vi "PH_PILS.set i Attr.vi"(2 "error in (no error)":errorcluster, 3 "DB Entry to read":string) -> (0 "error out":errorcluster, 1 "i Attr":T1={"Boolean"=[], "GUI Refs Exp. Shutters"={"1"=refnum, "2"=refnum, "3"=refnum, "4"=refnum}, "Tristate2Run GUI Refs"=[], "EO-Likes"=[], "Operation Mode"={"Operation Mode"=enum."unknown", "GUI"={"Ref State"=refnum, "Ref"=refnum}, "Servicemode"={"Tagname"="", "Status"=0}, "Labormode"={"Tagname"="", "Status"=0}, "Searchmode"={"Tagname"="", "Status"=0}, "Shotmode"={"Tagname"="", "Status"=0}}, "Submode"={"Submode"=enum."unknown", "GUI"={"Ref State"=refnum, "Ref"=refnum}, "Submode"={"Tagname"="", "Status"=0}}, "Experiment"={"Experiment"=enum."unknown", "GUI"={"Ref State"=refnum, "Ref"=refnum}, "intern"={"Tagname"="", "Status"=0}, "Exp 4"={"Tagname"="", "Status"=0}, "Exp 3"={"Tagname"="", "Status"=0}, "Exp 2"={"Tagname"="", "Status"=0}, "Exp 1"={"Tagname"="", "Status"=0}}, "TristateNormal"=[], "Door Tags"=[], "GUIlessTags"=[], "Beamline GUI Refs"=[], "Special Boolean"=[], "Laserpower"=[], "Shutter"=[], "Tristate EO Like"=[], "PP"=[], "Switch Knobs"=[], "Latch Knob GUI Refs"=[], "FailureCounter"=0, "Enabled Status"={"Laser"=0, "PreAmp"=0, "MainAmp"=0}, "Mercury"=refnum, "Instance Rods"="N/A", "Logfile"=path "", "Beckhoff-Instance Internal"="", "Beckhoff-Instance External"="", "Enabling Rights"=[]})   [LabVIEW 2014, in "PH_PILS.lvlib"]
doc: "This VI sets attributes."
uses:
  PH_PILS.lvlib
  PH_PILS.i attribute.ctl
  PH_PILS.Operation Mode.ctl
  PH_PILS.Submode.ctl
  PH_Common/PH_Common.lvlib
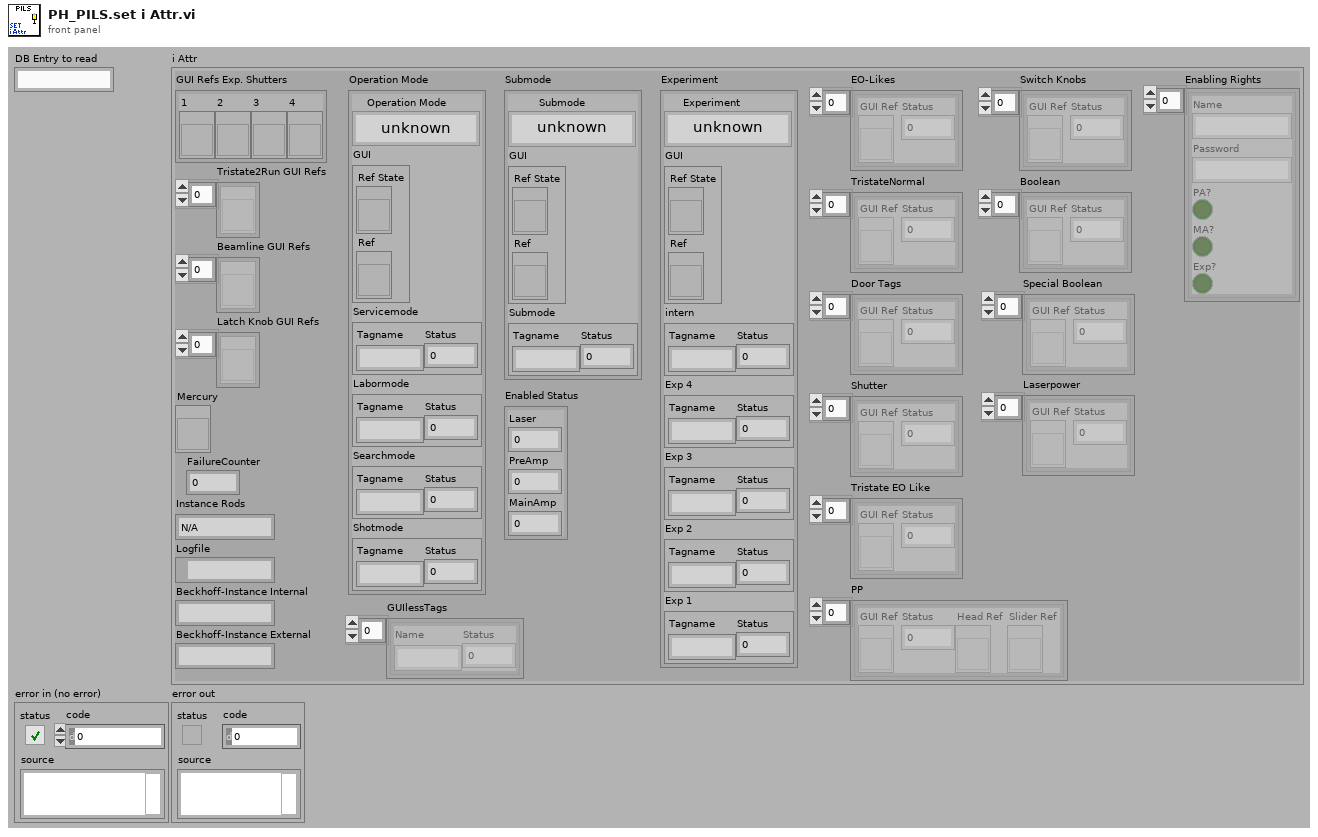
[diagram p1: front panel]
types:
  T1 = typedef "PH_PILS.lvlib/PH_PILS.i attribute.ctl" = cluster{"Boolean":cluster{"GUI Ref":refnum<vi>, "Status":i32}[], "GUI Refs Exp. Shutters":cluster{"1":refnum<vi>, "2":refnum<vi>, "3":refnum<vi>, "4":refnum<vi>}, "Tristate2Run GUI Refs":refnum<vi>[], "EO-Likes":cluster{"GUI Ref":refnum<vi>, "Status":i32}[], "Operation Mode":cluster{"Operation Mode":T2, "GUI":cluster{"Ref State":refnum<vi>, "Ref":refnum<vi>}, "Servicemode":cluster{"Tagname":string, "Status":i32}, "Labormode":cluster{"Tagname":string, "Status":i32}, "Searchmode":cluster{"Tagname":string, "Status":i32}, "Shotmode":cluster{"Tagname":string, "Status":i32}}, "Submode":cluster{"Submode":T3, "GUI":cluster{"Ref State":refnum<vi>, "Ref":refnum<vi>}, "Submode":cluster{"Tagname":string, "Status":i32}}, "Experiment":cluster{"Experiment":enum16{"unknown", "intern", "4 (Z6)", "3", "2", "1"}, "GUI":cluster{"Ref State":refnum<vi>, "Ref":refnum<vi>}, "intern":cluster{"Tagname":string, "Status":i32}, "Exp 4":cluster{"Tagname":string, "Status":i32}, "Exp 3":cluster{"Tagname":string, "Status":i32}, "Exp 2":cluster{"Tagname":string, "Status":i32}, "Exp 1":cluster{"Tagname":string, "Status":i32}}, "TristateNormal":cluster{"GUI Ref":refnum<vi>, "Status":i32}[], "Door Tags":cluster{"GUI Ref":refnum<vi>, "Status":i32}[], "GUIlessTags":cluster{"Name":string, "Status":i32}[], "Beamline GUI Refs":refnum<vi>[], "Special Boolean":cluster{"GUI Ref":refnum<vi>, "Status":i32}[], "Laserpower":cluster{"GUI Ref":refnum<vi>, "Status":i32}[], "Shutter":cluster{"GUI Ref":refnum<vi>, "Status":i32}[], "Tristate EO Like":cluster{"GUI Ref":refnum<vi>, "Status":i32}[], "PP":cluster{"GUI Ref":refnum<vi>, "Status":i32, "Head Ref":refnum<vi>, "Slider Ref":refnum<vi>}[], "Switch Knobs":cluster{"GUI Ref":refnum<vi>, "Status":i32}[], "Latch Knob GUI Refs":refnum<vi>[], "FailureCounter":i32, "Enabled Status":cluster{"Laser":i32, "PreAmp":i32, "MainAmp":i32}, "Mercury":refnum<vi>, "Instance Rods":string, "Logfile":path, "Beckhoff-Instance Internal":string, "Beckhoff-Instance External":string, "Enabling Rights":cluster{"Name":string, "Password":string, "PA?":bool, "MA?":bool, "Exp?":bool}[]}
  T2 = typedef "PH_PILS.lvlib/PH_PILS.Operation Mode.ctl" = enum16{"unknown", "Service", "Labor", "Search", "Shot"}
  T3 = typedef "PH_PILS.lvlib/PH_PILS.Submode.ctl" = enum16{"unknown", "HV-Normal", "HV-Test"}
  T4 = cluster{"Name":string, "Password":string, "PA?":bool, "MA?":bool, "Exp?":bool}
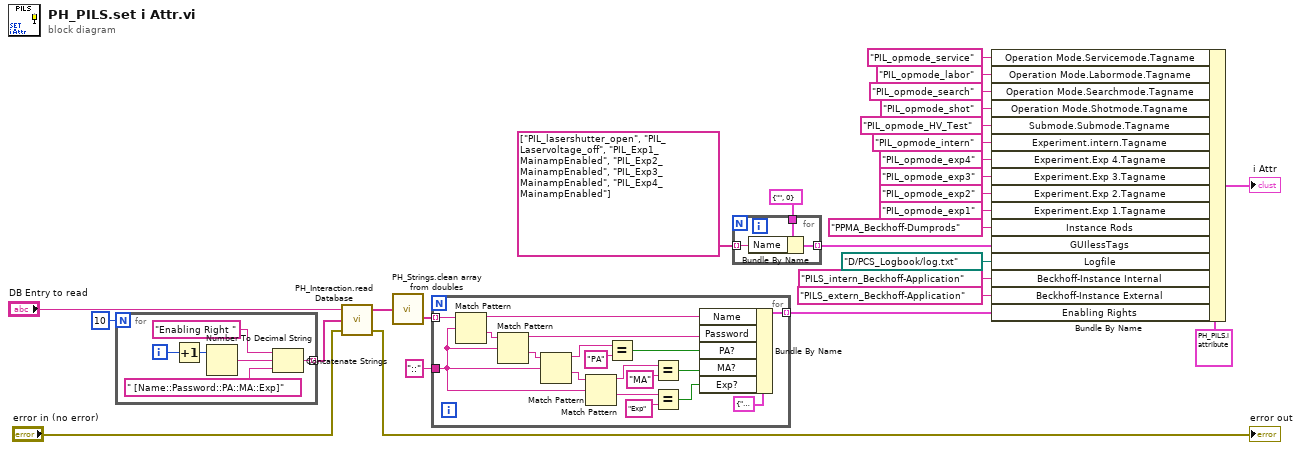
[diagram p0: block diagram]
diagram:
  n1 = for {
    N: 10 -> [_]
    tunnel: [w29] -> w4 mode=indexing
    i -> [w33]
    n2 = Increment(x=w33) -> (x+1=w32:i32)
    n3 = Number To Decimal String(number=w32) -> (decimal integer string=w34:string)  [unwired: 1 in]
    n4 = Concatenate Strings("Enabling Right ", w34, " [Name::Password::PA::MA::Exp]") -> (w29:string)
  }
  n5 = call "PH_Interaction.read Database.vi"("error in (no error)"="error in (no error)", "Strings to search for"=w4, "DB Entry to read"="DB Entry to read") -> ("error out"=→"error out":errorcluster, "Values"=w3:string[])  [unwired: 1 in]
  n6 = call "PH_Strings.clean array from doubles.vi"("Array Input"=w3) -> ("Cleaned Array Output"=w2:string[])  [unwired: 1 out]
  n7 = for {
    tunnel: w2 -> [w51] mode=indexing
    tunnel: [w52] -> w1 mode=indexing
    tunnel: "::" ("regular expression") -> [w42]
    n8 = Match Pattern(string=w51, regular expression=w42) -> (before substring=w50:string, after substring=w49:string)  [unwired: 1 in, 2 out]
    n9 = Match Pattern(string=w49, regular expression=w42) -> (before substring=w48:string, after substring=w47:string)  [unwired: 1 in, 2 out]
    n10 = Match Pattern(string=w47, regular expression=w42) -> (before substring=w46:string, after substring=w43:string)  [unwired: 1 in, 2 out]
    n11 = Match Pattern(string=w43, regular expression=w42) -> (before substring=w40:string, after substring=w38:string)  [unwired: 1 in, 2 out]
    n12 = Equal?(x=w46, y="PA") -> (x = y?=w44:bool)
    n13 = Equal?(x=w40, y="MA") -> (x = y?=w41:bool)
    n14 = Equal?(x=w38, y="Exp") -> (x = y?=w37:bool)
    n15 = Bundle By Name(cluster=T4 {"Name"="", "Password"="", "PA?"=FALSE, "MA?"=FALSE, "Exp?"=FALSE} ("Cluster"), "Name"=w50, "Password"=w48, "PA?"=w44, "MA?"=w41, "Exp?"=w37) -> (w52:T4)
  }
  n16 = for {
    tunnel: cluster{"Name":string, "Status":i32} {"Name"="", "Status"=0} ("Tag") -> [w55]
    tunnel: string[] ["PIL_lasershutter_open", "PIL_Laservoltage_off", "PIL_Exp1_MainampEnabled", "PIL_Exp2_MainampEnabled", "PIL_Exp3_MainampEnabled", "PIL_Exp4_MainampEnabled"] -> [w54] mode=indexing
    tunnel: [w53] -> w16 mode=indexing
    n17 = Bundle By Name(cluster=w55, "Name"=w54) -> (w53:cluster{"Name":string, "Status":i32})
  }
  n18 = Bundle By Name(cluster=T1 {"Boolean"=[], "GUI Refs Exp. Shutters"={"1"=refnum, "2"=refnum, "3"=refnum, "4"=refnum}, "Tristate2Run GUI Refs"=[], "EO-Likes"=[], "Operation Mode"={"Operation Mode"=enum."unknown", "GUI"={"Ref State"=refnum, "Ref"=refnum}, "Servicemode"={"Tagname"="", "Status"=0}, "Labormode"={"Tagname"="", "Status"=0}, "Searchmode"={"Tagname"="", "Status"=0}, "Shotmode"={"Tagname"="", "Status"=0}}, "Submode"={"Submode"=enum."unknown", "GUI"={"Ref State"=refnum, "Ref"=refnum}, "Submode"={"Tagname"="", "Status"=0}}, "Experiment"={"Experiment"=enum."unknown", "GUI"={"Ref State"=refnum, "Ref"=refnum}, "intern"={"Tagname"="", "Status"=0}, "Exp 4"={"Tagname"="", "Status"=0}, "Exp 3"={"Tagname"="", "Status"=0}, "Exp 2"={"Tagname"="", "Status"=0}, "Exp 1"={"Tagname"="", "Status"=0}}, "TristateNormal"=[], "Door Tags"=[], "GUIlessTags"=[], "Beamline GUI Refs"=[], "Special Boolean"=[], "Laserpower"=[], "Shutter"=[], "Tristate EO Like"=[], "PP"=[], "Switch Knobs"=[], "Latch Knob GUI Refs"=[], "FailureCounter"=0, "Enabled Status"={"Laser"=0, "PreAmp"=0, "MainAmp"=0}, "Mercury"=refnum, "Instance Rods"="N/A", "Logfile"=path "", "Beckhoff-Instance Internal"="", "Beckhoff-Instance External"="", "Enabling Rights"=[]} ("i Attr"), "Operation Mode.Servicemode.Tagname"="PIL_opmode_service", "Operation Mode.Labormode.Tagname"="PIL_opmode_labor", "Operation Mode.Searchmode.Tagname"="PIL_opmode_search", "Operation Mode.Shotmode.Tagname"="PIL_opmode_shot", "Submode.Submode.Tagname"="PIL_opmode_HV_Test", "Experiment.intern.Tagname"="PIL_opmode_intern", "Experiment.Exp 4.Tagname"="PIL_opmode_exp4", "Experiment.Exp 3.Tagname"="PIL_opmode_exp3", "Experiment.Exp 2.Tagname"="PIL_opmode_exp2", "Experiment.Exp 1.Tagname"="PIL_opmode_exp1", "Instance Rods"="PPMA_Beckhoff-Dumprods", "GUIlessTags"=w16, "Logfile"=path "D:/PCS_Logbook/log.txt", "Beckhoff-Instance Internal"="PILS_intern_Beckhoff-Application", "Beckhoff-Instance External"="PILS_extern_Beckhoff-Application", "Enabling Rights"=w1) -> (→"i Attr":T1)
